vi "Get_LibName_From_QualName.vi"(11 "QualifiedName":string) -> (3 "ProperlyFormattedLibraryName":string)   [LabVIEW 2020]
uses:
  e:/builds/penguin/labview/branches/2020/dev/dist/resource/NationalInstruments.LabVIEW.Generator.dll
  resource/NationalInstruments.LabVIEW.Generator.dll
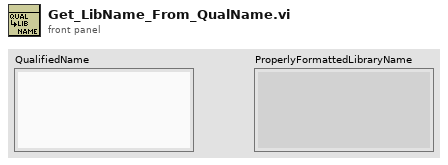
[diagram p1: front panel]
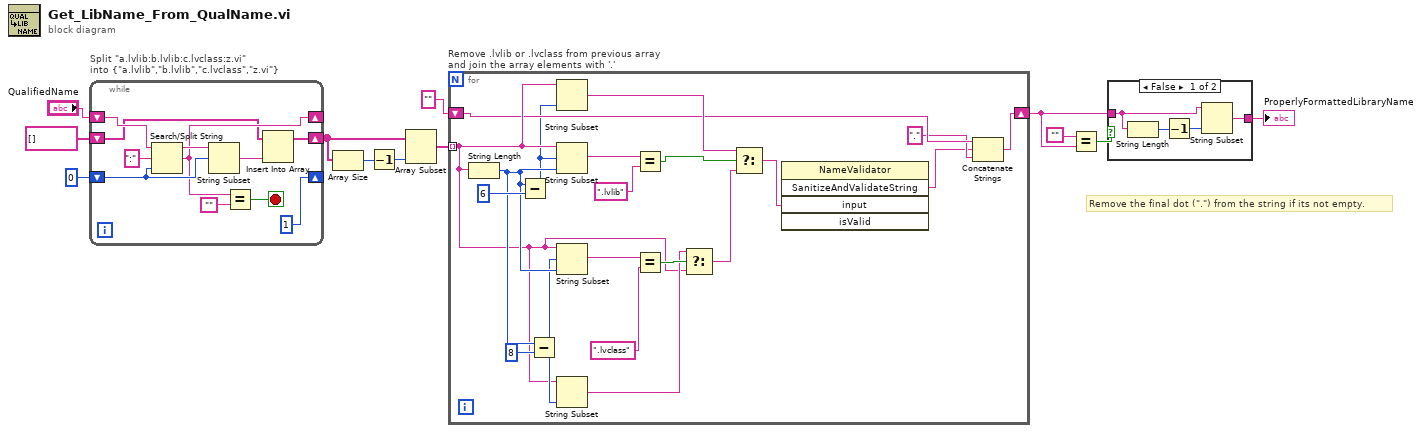
[diagram p0: block diagram]
diagram:
  # "Remove the final dot (\".\") from the string if its not empty."
  n1 = while "Split \"a.lvlib:b.lvlib:c.lvclass:z.vi\" \ninto {\"a.lvlib\",\"b.lvlib\",\"c.lvclass\",\"z.vi\"}" {
    shift-right: [w14] -> w9
    shift-left: string[] [] -> [w16]
    shift-right: [1] -> _
    shift-left: 0 -> [w20]
    shift-right: [w19] -> _
    shift-left: "QualifiedName" -> [w23]
    stop <- w17 stop-if-true
    n2 = Search/Split String(string=w23, search string/char (-)=":", offset (0)=w20) -> (substring before match=w21:string, match + rest of string=w19:string)  [unwired: 1 out]
    n3 = String Subset(string=w21, offset (0)=w20) -> (substring=w15:string)  [unwired: 1 in]
    n4 = Equal?(x=w19, y="") -> (x = y?=w17:bool)
    n5 = Insert Into Array(array=w16, new element=w15) -> (w14:string[])  [unwired: 1 in]
  }
  n6 = Array Size(array=w9) -> (size(s)=w8:i32)
  n7 = Decrement(x=w8) -> (x-1=w7:i32)
  n8 = Array Subset(array=w9, length=w7) -> (w6:string[])  [unwired: 1 in]
  n9 = for "Remove .lvlib or .lvclass from previous array and join the array elements with '.'" {
    tunnel: w6 -> [w31] mode=indexing
    shift-right: [w27] -> w1
    shift-left: "" ("match + rest of string") -> [w29]
    n10 = String Length(string=w31) -> (length=w37:i32)
    n11 = Subtract(x=w37, y=6) -> (x-y=w26:i32)
    n12 = Subtract(x=w37, y=8) -> (x-y=w35:i32)
    n13 = String Subset(string=w31, length (rest)=w26) -> (substring=w33:string)  [unwired: 1 in]
    n14 = String Subset(string=w31, offset (0)=w26, length (rest)=w37) -> (substring=w42:string)
    n15 = String Subset(string=w31, offset (0)=w35, length (rest)=w37) -> (substring=w39:string)
    n16 = String Subset(string=w31, length (rest)=w35) -> (substring=w32:string)  [unwired: 1 in]
    n17 = Equal?(x=w42, y=".lvlib") -> (x = y?=w34:bool)
    n18 = Equal?(x=w39, y=".lvclass") -> (x = y?=w36:bool)
    n19 = Select(t=w32, s=w36, f=w31) -> (s? t:f=w30:string)
    n20 = Select(t=w33, s=w34, f=w30) -> (s? t:f=w25:string)
    n21 = invoke class="NameValidator" method="SanitizeAndValidateString"("input"=w25) -> ("SanitizeAndValidateString"=w24:string)  [unwired: 4 in, 4 out]
    n22 = Concatenate Strings(w29, w24, "." ("string")) -> (w27:string)
  }
  n23 = Equal?(x="", y=w1) -> (x = y?=w3:bool)
  n24 = case shown="False" w3 {
    tunnel: [w44 w48] -> w2
    tunnel: w1 -> [w46 w48]
    frame False {
      n25 = String Length(string=w46) -> (length=w47:i32)
      n26 = Decrement(x=w47) -> (x-1=w45:i32)
      n27 = String Subset(string=w46, length (rest)=w45) -> (substring=w44:string)  [unwired: 1 in]
    }
    frame True {
    }
  }
  "ProperlyFormattedLibraryName" <- w2
